vi "Stop.vi"(8 "error in (no error)":errorcluster, 10 "Message in":refnum<class "StopMessage.lvclass">, 11 "DAQMH121119OrcaFlash in":refnum<class "DAQOrcaFlash.lvclass">) -> (0 "error out":errorcluster, 3 "DAQMH121119OrcaFlash out":refnum<class "DAQOrcaFlash.lvclass">)   [LabVIEW 2012, in "DAQOrcaFlash.lvclass"]
doc: "This member function is called when the statemachine in the run.vi receives an 'stop' command. It relays the message to all observers of the component.\n\nOverride this member function in your derived class if you need additional stop functionality (but don't forget to call the parent method)."
uses:
  DAQOrcaFlash.lvclass
  <vilib>/Distrio/Murmex/StopMessage/StopMessage.lvclass
  <vilib>/Distrio/Murmex/Murmex/Murmex.lvclass
  DAQOrcaFlash.lvclass/DAQOrcaFlash.ctl
  imaging_mode.ctl
panel:
  # "This method is called when the STOP\ntrigger is sent. \n\nOverride this method when your component needs to\nrespond to this trigger. \n\nCall parent for proper implementation"
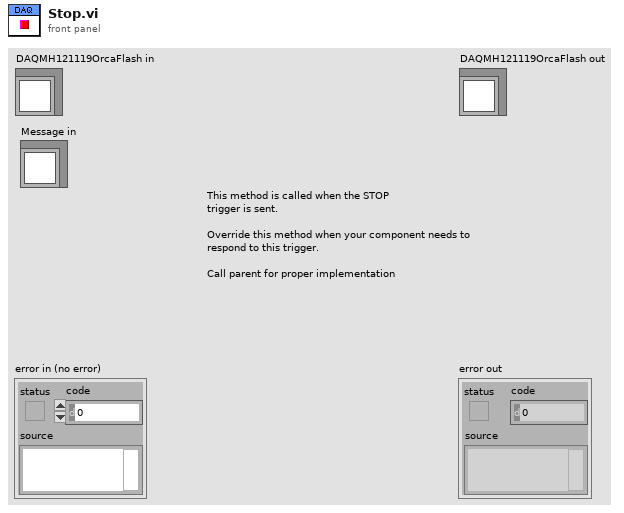
[diagram p1: front panel]
types:
  T1 = cluster{"Mode":u32, "Polarity":u32, "Period":dbl, "Delay":dbl}
  T2 = typedef "DAQOrcaFlash.lvclass/imaging_mode.ctl" = enum16{"focus mode", "single sweep"}
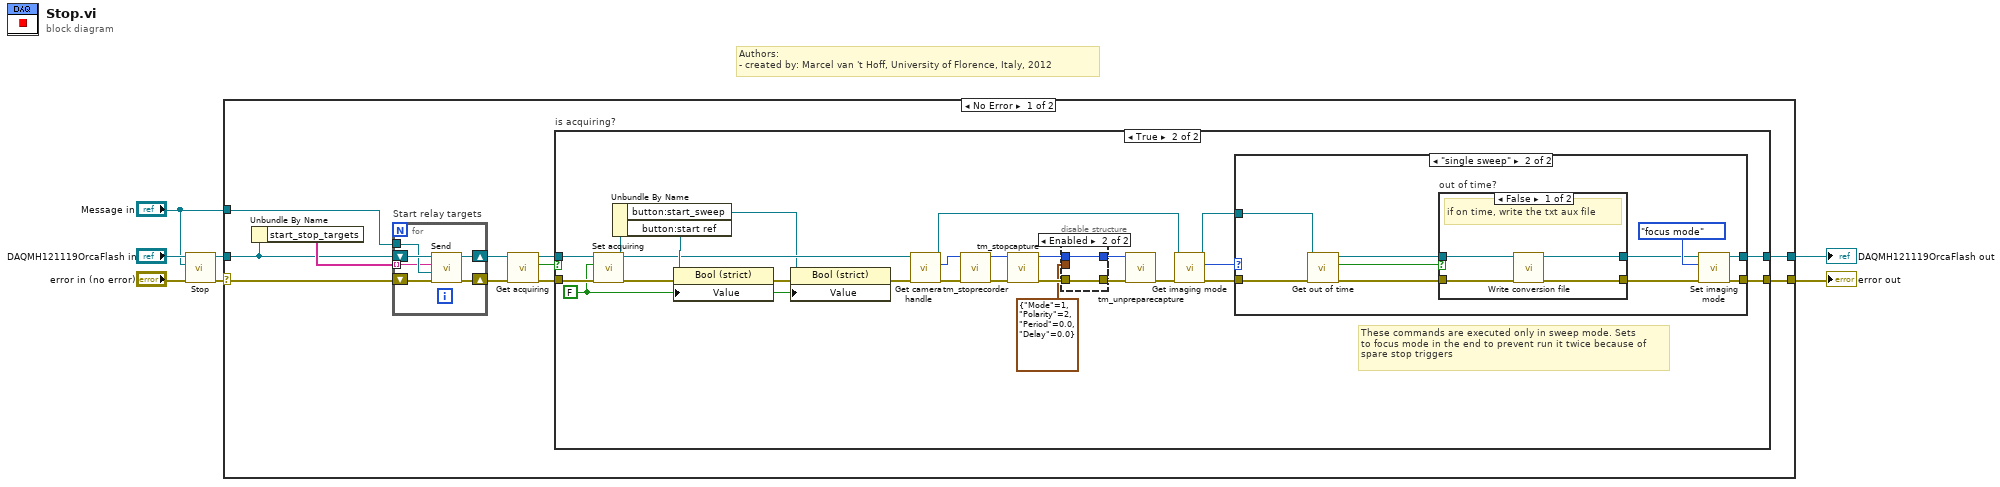
[diagram p0: block diagram]
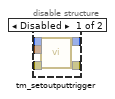
[diagram p5: hidden frame]
diagram:
  # "Authors: \n- created by: Marcel van 't Hoff, University of Florence, Italy, 2012"
  n1 = call-parent "Stop.vi"("error in (no error)"="error in (no error)", "Message in"="Message in", "Murmex in"="DAQMH121119OrcaFlash in") -> ("error out"=w5:errorcluster, "Murmex out"=w2:refnum<class "DAQOrcaFlash.lvclass">)  [unwired: 7 in]
  n2 = case shown="No Error" w5 {
    selector: w5 -> [w14 w77]
    tunnel: [w9 w77] -> w4
    tunnel: [w8 w78] -> w3
    tunnel: w2 -> [w12 w78]
    tunnel: "Message in" -> [w10 _]
    frame No Error {
      n3 = Unbundle By Name(w12) -> ("start_stop_targets"=w15:string[])
      n4 = for "Start relay targets" {
        shift-right: [w24] -> w13
        shift-left: w14 -> [w23]
        tunnel: w10 -> [w21]
        tunnel: w15 -> [w20] mode=indexing
        shift-right: [w19] -> w11
        shift-left: w12 -> [w22]
        n5 = call <vilib>:"Send.vi"("error in (no error)"=w23, "Message"=w21, "recipient"=w20, "Murmex in"=w22) -> ("error out"=w24:errorcluster, "Murmex out"=w19:refnum<class "DAQOrcaFlash.lvclass">)  [unwired: 6 in]
      }
      n6 = call "Get acquiring.vi"("error in (no error)"=w13, "DAQMH121119OrcaFlash in"=w11) -> ("error out"=w17:errorcluster, "is acquiring?"=w16:bool, "DAQMH121119OrcaFlash out"=w18:refnum<class "DAQOrcaFlash.lvclass">)  [unwired: 7 in]
      n7 = case "is acquiring?" shown="True" w16 {
        tunnel: [w25 w31] -> w8
        tunnel: [w26 w32] -> w9
        tunnel: w18 -> [w25 w48]
        tunnel: w17 -> [w26 w47]
        frame False {
        }
        frame True {
          w43 = FALSE ("is acquiring?")
          # "These commands are executed only in sweep mode. Sets\nto focus mode in the end to prevent run it twice because of \nspare stop triggers"
          n8 = call "Set acquiring.vi"("error in (no error)"=w47, "is acquiring?"=w43, "DAQMH121119OrcaFlash in"=w48) -> ("error out"=w50:errorcluster, "DAQMH121119OrcaFlash out"=w49:refnum<class "DAQOrcaFlash.lvclass">)  [unwired: 7 in]
          n9 = Unbundle By Name(w49) -> ("button:start_sweep"=w46:refnum<vi>, "button:start ref"=w51:refnum<vi>)
          n10 = property class="Bool (strict)"(reference=w51, error in=w50, "Value"=w43) -> (error out=w45:errorcluster)  [unwired: 1 out]
          n11 = property class="Bool (strict)"(reference=w46, error in=w45, "Value"=w43) -> (error out=w44:errorcluster)  [unwired: 1 out]
          n12 = call "Get camera handle.vi"("error in (no error)"=w44, "DAQMH121119OrcaFlash in"=w49) -> ("error out"=w42:errorcluster, "cam handle"=w41:u32, "DAQMH121119OrcaFlash out"=w29:refnum<class "DAQOrcaFlash.lvclass">)  [unwired: 7 in]
          n13 = call <userlib>:"tm_stoprecorder.vi"("error in (no error)"=w42, "Handle in"=w41) -> ("error out"=w39:errorcluster, "Handle out"=w40:u32)  [unwired: 8 in]
          n14 = call <userlib>:"tm_stopcapture.vi"("error in (no error)"=w39, "Handle in"=w40) -> ("error out"=w36:errorcluster, "Handle out"=w38:u32)  [unwired: 8 in]
          n15 = disable-structure shown="Enabled" {
            disable-tunnel: w38 -> [w74 w75]
            disable-tunnel: [w73 w75] -> w37
            disable-tunnel: w36 -> [w72 w76]
            disable-tunnel: [w71 w76] -> w34
            disable-tunnel: T1 {"Mode"=1, "Polarity"=2, "Period"=0.0, "Delay"=0.0} ("Parameters") -> [w70 _]
            frame Disabled {
              n16 = call <userlib>:"tm_setoutputtrigger.vi"("error in (no error)"=w72, "Parameters"=w70, "Handle in"=w74) -> ("error out"=w71:errorcluster, "Handle out"=w73:u32)  [unwired: 7 in]
            }
            frame Enabled {
            }
          }
          n17 = call <userlib>:"tm_unpreparecapture.vi"("error in (no error)"=w34, "Handle in"=w37) -> ("error out"=w33:errorcluster)  [unwired: 8 in, 1 out]
          n18 = call "Get imaging mode.vi"("error in (no error)"=w33, "DAQMH121119OrcaFlash in"=w29) -> ("error out"=w30:errorcluster, "imaging mode"=w27:T2, "DAQMH121119OrcaFlash out"=w28:refnum<class "DAQOrcaFlash.lvclass">)  [unwired: 7 in]
          n19 = case shown="\"single sweep\"" w27 {
            tunnel: w30 -> [w52 w58]
            tunnel: [w52 w63] -> w32
            tunnel: [w53 w62] -> w31
            tunnel: w28 -> [w53 w57]
            frame "focus mode", Default {
            }
            frame "single sweep" {
              n20 = call-dynamic "Get out of time.vi"("error in (no error)"=w58, "DAQOrcaFlash in"=w57) -> ("error out"=w54:errorcluster, "out of time?"=w56:bool, "DAQOrcaFlash out"=w55:refnum<class "DAQOrcaFlash.lvclass">)  [unwired: 7 in]
              n21 = case "out of time?" shown="False" w56 {
                tunnel: w54 -> [w67 w68]
                tunnel: [w66 w68] -> w60
                tunnel: w55 -> [w65 w69]
                tunnel: [w64 w69] -> w59
                frame False {
                  # "if on time, write the txt aux file"
                  n22 = call-dynamic "Write conversion file.vi"("error in (no error)"=w67, "DAQOrcaFlash in"=w65) -> ("error out"=w66:errorcluster, "DAQOrcaFlash out"=w64:refnum<class "DAQOrcaFlash.lvclass">)  [unwired: 8 in]
                }
                frame True {
                  # "if out of time do nothing"
                }
              }
              n23 = call "Set imaging mode.vi"("error in (no error)"=w60, "imaging mode"=imaging_mode."focus mode", "DAQMH121119OrcaFlash in"=w59) -> ("error out"=w63:errorcluster, "DAQMH121119OrcaFlash out"=w62:refnum<class "DAQOrcaFlash.lvclass">)  [unwired: 7 in]
            }
          }
        }
      }
    }
    frame Error {
    }
  }
  "error out" <- w4
  "DAQMH121119OrcaFlash out" <- w3
